vi "SHTBoxConfigJson.vi"(8 "error in (no error)":errorcluster, 11 "JSON string":string) -> (0 "error out":errorcluster, 3 "value":T1)   [LabVIEW 2018]
panel:
  in  "boxConfig":T1
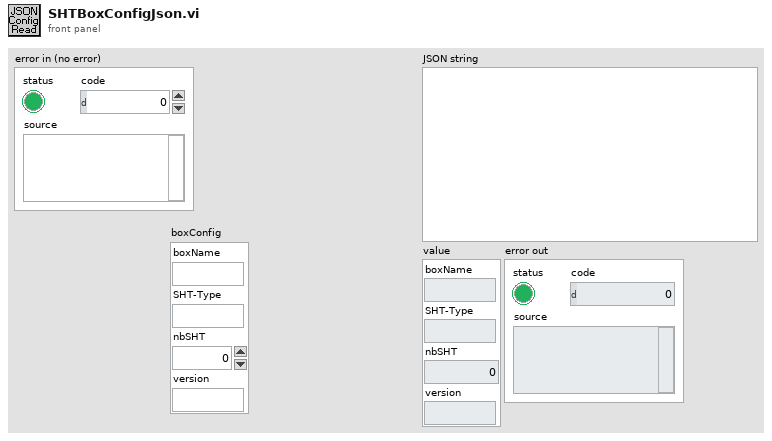
[diagram p1: front panel]
types:
  T1 = cluster{"boxName":string, "SHT-Type":string, "nbSHT":dbl, "version":string}
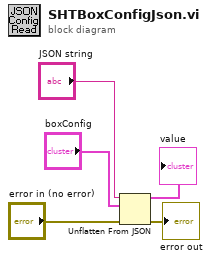
[diagram p0: block diagram]
diagram:
  n1 = Unflatten From JSON(JSON string="JSON string", type and defaults="boxConfig", error in (no error)="error in (no error)") -> (value=→"value":T1, error out=→"error out":errorcluster)  [unwired: 4 in]
